vi "Set Letter Time Core.vi"(8 "error in (no error)":errorcluster, 9 "Time":dbl[unit], 10 "Letter":string, 11 "CS++PPG in":refnum<class "CS++PPG.lvclass">) -> (0 "error out":errorcluster, 3 "CS++PPG out":refnum<class "CS++PPG.lvclass">)   [LabVIEW 2016, in "CS++PPG.lvlib" / "CS++PPG.lvclass"]
doc: "This VI sets a new time value for a given letter of the timing pattern. This should also work while the pulsed pattern generator is running."
uses:
  CS++PPG.lvclass
  CS++PPG.lvclass/CS++PPG.ctl
  CSPP_Core/Libraries/Utilities/CS++Utilities.lvlib
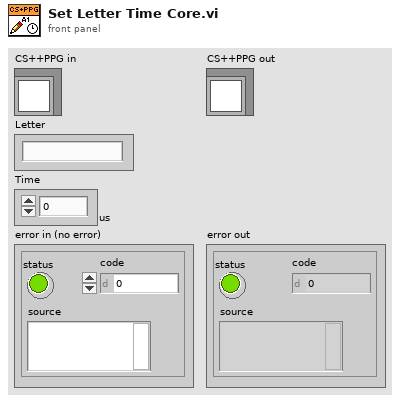
[diagram p1: front panel]
types:
  T1 = cluster{"TriggerCondition":i32, "TimeTable":dbl[], "ChannelTable":string[]}[]
  T2 = cluster{"TriggerCondition":i32, "TimeTable":dbl[], "ChannelTable":string[]}
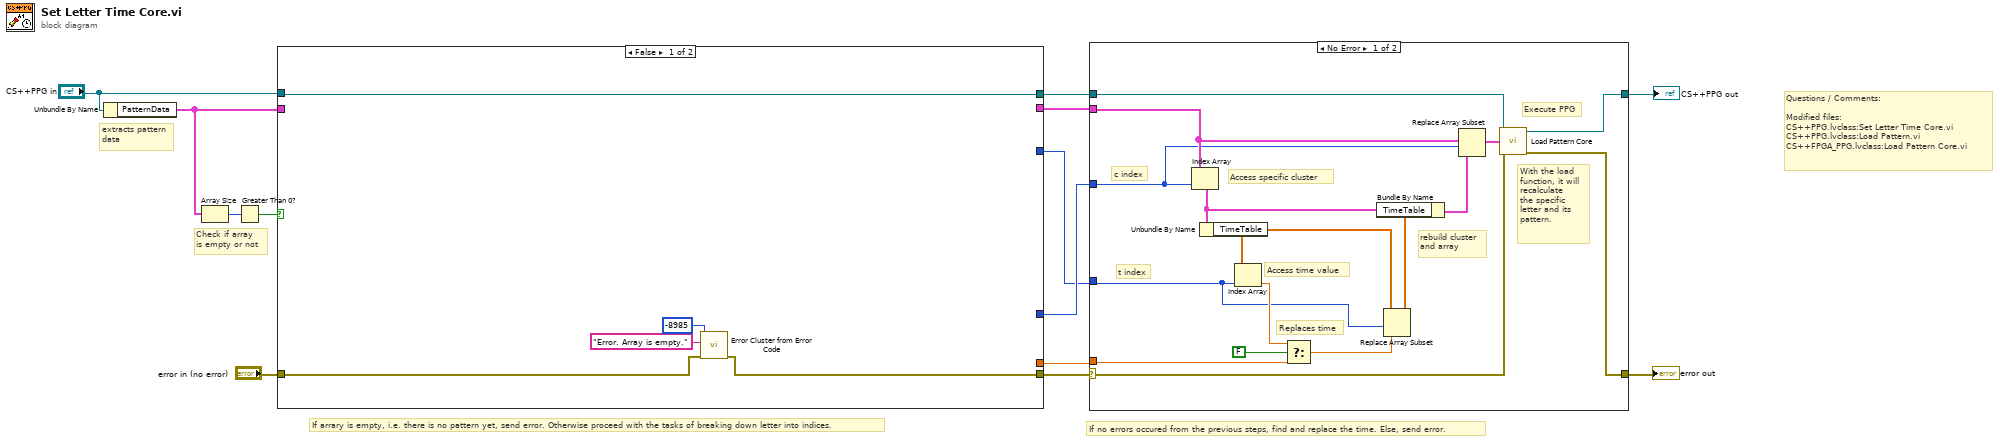
[diagram p0: block diagram]
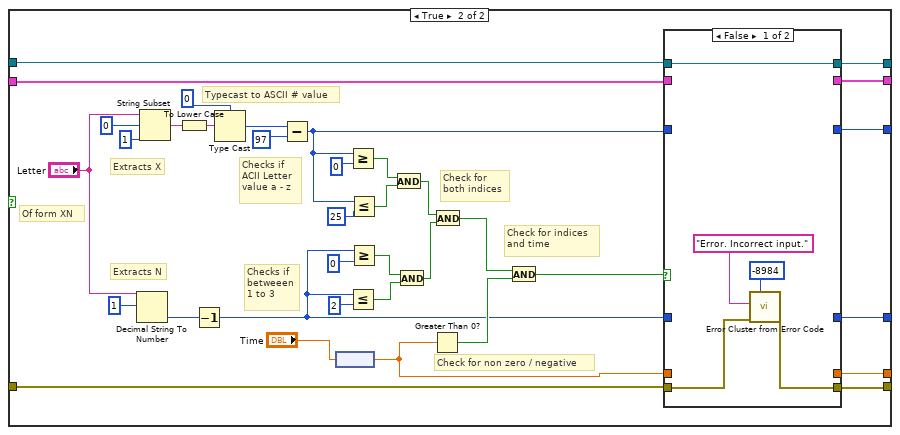
[diagram p2: hidden frame]
diagram:
  # "Questions / Comments:\n\nModified files:\nCS++PPG.lvclass:Set Letter Time Core.vi\nCS++PPG.lvclass:Load Pattern.vi\nCS++FPGA_PPG.lvclass:Load Pattern Core.vi"
  # "If no errors occured from the previous steps, find and replace the time. Else, send error."
  # "If arrary is empty, i.e. there is no pattern yet, send error. Otherwise proceed with the tasks of breaking down letter into indices."
  # "extracts pattern\ndata"
  # "Check if array\nis empty or not"
  n1 = Unbundle By Name("CS++PPG in") -> ("PatternData"=w7:T1)
  n2 = Array Size(array=w7) -> (size(s)=w11:i32)
  n3 = Greater Than 0?(x=w11) -> (x > 0?=w10:bool)
  n4 = case shown="False" w10 {
    tunnel: "error in (no error)" -> [w17 w33]
    tunnel: [w16 w30] -> w6
    tunnel: "CS++PPG in" -> [w18 w31]
    tunnel: w7 -> [_ w27]
    tunnel: [_ w29] -> w5
    tunnel: [w18 w28] -> w4
    tunnel: [_ w26] -> w3
    tunnel: [_ w23] -> w2
    tunnel: [_ w22] -> w1
    frame False {
      n5 = call "Error Cluster from Error Code.vi"("Error In"=w17, "Error Message (\"\")"="Error. Array is empty." ("Error Message (\"\")"), "Error Code (0)"=-8985) -> ("Error Out"=w16:errorcluster)  [unwired: 8 in]
    }
    frame True {
      # "Check for indices\nand time"
      # "Check for non zero / negative"
      # "Of form XN"
      # "Check for\nboth indices"
      # "Checks if \nbetweeen\n1 to 3"
      # "Checks if\nACII Letter \nvalue a - z"
      # "Typecast to ASCII # value"
      # "Extracts X"
      # "Extracts N"
      n6 = Decimal String To Number(string="Letter", offset=1) -> (number=w25:i32)  [unwired: 1 in, 1 out]
      n7 = String Subset(string="Letter", offset (0)=0, length (rest)=1 ("length (rest)")) -> (substring=w43:string)
      n8 = To Lower Case(string=w43) -> (all lower case string=w42:string)
      n9 = Decrement(x=w25) -> (x-1=w19:i32)
      n10 = Type Cast(type=u8 0 ("offset (0)"), x=w42) -> (*(type *) &x=w44:u8)
      n11 = Subtract(x=w44, y=97) -> (x-y=w24:i32)
      n12 = node("Time") -> (w21:dbl)
      n13 = Greater Or Equal?(x=w24, y=0) -> (x >= y?=w38:bool)
      n14 = Less Or Equal?(x=w19, y=2) -> (x <= y?=w50:bool)
      n15 = Less Or Equal?(x=w24, y=25) -> (x <= y?=w36:bool)
      n16 = Greater Or Equal?(x=w19, y=0) -> (x >= y?=w51:bool)
      n17 = And(x=w38, y=w36) -> (x .and. y?=w37:bool)
      n18 = And(x=w51, y=w50) -> (x .and. y?=w46:bool)
      n19 = Greater Than 0?(x=w21) -> (x > 0?=w35:bool)
      n20 = And(x=w37, y=w46) -> (x .and. y?=w34:bool)
      n21 = And(x=w34, y=w35) -> (x .and. y?=w32:bool)
      n22 = case shown="False" w32 {
        tunnel: [w57 w65] -> w30
        tunnel: w33 -> [w58 w65]
        tunnel: w31 -> [w59 w63]
        tunnel: [w59 w63] -> w28
        tunnel: w21 -> [_ w64]
        tunnel: [_ w64] -> w29
        tunnel: w27 -> [_ w62]
        tunnel: [_ w62] -> w26
        tunnel: w19 -> [_ w60]
        tunnel: w24 -> [_ w61]
        tunnel: [_ w61] -> w22
        tunnel: [_ w60] -> w23
        frame False {
          n23 = call "Error Cluster from Error Code.vi"("Error In"=w58, "Error Message (\"\")"="Error. Incorrect input." ("Error Message (\"\")"), "Error Code (0)"=-8984) -> ("Error Out"=w57:errorcluster)  [unwired: 8 in]
        }
        frame True {
          # "If the indices exist,\nand time is non zero\nand positive, then the\nvalues may be sent\nthrough to the next \nphase of replacing\nand setting the time.\nOtherwise send error."
          # "Passes time index"
          # "Passes cluster index"
        }
      }
    }
  }
  n24 = case shown="No Error" w6 {
    selector: w6 -> [w75 w83]
    tunnel: [w70 w83] -> w13
    tunnel: [w71 w82] -> w12
    tunnel: w4 -> [w76 w82]
    tunnel: w5 -> [w68 _]
    tunnel: w3 -> [w69 _]
    tunnel: w1 -> [w67 _]
    tunnel: w2 -> [w66 _]
    frame No Error {
      # "With the load\nfunction, it will\nrecalculate \nthe specific \nletter and its \npattern."
      # "rebuild cluster\nand array"
      # "c index"
      # "t index"
      # "Access time value"
      # "Execute PPG"
      # "Replaces time"
      # "Access specific cluster"
      n25 = Index Array(array=w69, index=w66) -> (element=w79:T2)
      n26 = Unbundle By Name(w79) -> ("TimeTable"=w81:dbl[])
      n27 = Index Array(array=w81, index=w67) -> (element=w74:dbl)
      n28 = Select(t=w74, s=FALSE, f=w68) -> (s? t:f=w72:dbl)
      n29 = Replace Array Subset(array=w81, new element=w72, index=w67) -> (w80:dbl[])
      n30 = Bundle By Name(cluster=w79, "TimeTable"=w80) -> (w78:T2)
      n31 = Replace Array Subset(array=w69, new element=w78, index=w66) -> (w77:T1)
      n32 = call-dynamic "Load Pattern Core.vi"("error in (no error)"=w75, "PatternData"=w77, "CS++PPG in"=w76) -> ("error out"=w70:errorcluster, "CS++PPG out"=w71:refnum<class "CS++PPG.lvclass">)  [unwired: 7 in]
    }
    frame Error {
    }
  }
  "error out" <- w13
  "CS++PPG out" <- w12
